vi "Interpolate SMPS distribution.vi"(8 "method":i32(ring)=3 items=["nearest", "linear", "spline", "cubic Hermite", "Lagrange"], 9 "samples":i32=10000, 10 "SMPS Sizes":dbl[](array[numeric])=[105.5, 109.4, 113.4, 117.6, 121.9, 126.3, 131.0, 135.8, 140.7, 145.9, 151.2, 156.8, 162.5, 168.5, 174.7, 181.1, 187.7, 194.6, 201.7, 209.1, 216.7, 224.7, 232.9, 241.4, 250.3, 259.5, 269.0, 278.8, 289.0, 299.6, 310.6, 322.0, 333.8, 346.0, 358.7, 371.8, 385.4, 399.5, 414.2, 429.4, 445.1, 461.4, 478.3, 495.8, 514.0, 532.8, 552.3, 572.5, 593.5, 615.3, 637.8, 661.2, 685.4, 710.5, 736.5, 763.5, 791.5], 11 "Concentration":dbl[](array[numeric])=[0.0, 0.0, 0.0, 0.0, 0.0, 0.0, 0.0, 0.0, 0.0, 0.0, 0.0, 0.0, 0.0, 0.0, 0.0, 0.0, 0.0, 0.0, 0.0, 0.0, 0.0, 0.0, 0.0, 0.0, 0.0, 0.0, 0.0, 0.0, 0.0, 0.0, 0.0, 0.0, 0.0, 0.0, 0.0, 0.0, 0.0, 0.0, 0.00157646, 0.0185973, 0.0849944, 0.192093, 0.275242, 0.234884, 0.133371, 0.0469575, 0.0107273, 0.00146543, 9.21708e-05, 0.0, 0.0, 0.0, 0.0, 0.0, 0.0, 0.0, 0.0]) -> (1 "DeltaX":dbl=8.752859881644426e-05, 2 "xi used":dbl[](array[numeric]), 3 "yi":dbl[](array[numeric]))   [LabVIEW 2013]
doc: "Interpolates SMPS distribution according to the number of sizes needed"
uses:
  <vilib>/Analysis/1siggen.llb/Ramp Pattern by Samples.vi
  <vilib>/gmath/NI_Gmath.lvlib
  <vilib>/Analysis/NI_AALBase.lvlib
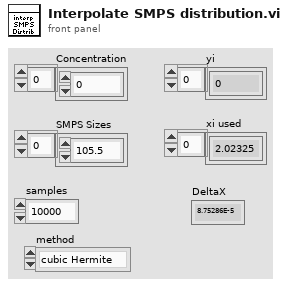
[diagram p1: front panel]
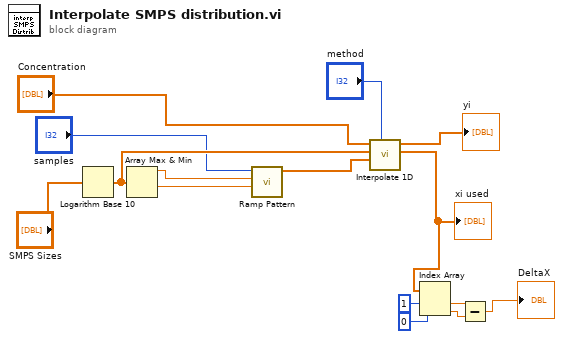
[diagram p0: block diagram]
diagram:
  n1 = Logarithm Base 10(1:"SMPS Sizes") -> (0:w13:dbl[])
  n2 = Array Max & Min(array=w13) -> (max value=w8:dbl, min value=w9:dbl)  [unwired: 2 out]
  n3 = call-poly <vilib>:"Ramp Pattern.vi"("start"=w9, "end"=w8, "samples"="samples") -> ("Ramp Pattern"=w11:dbl[])  [unwired: 7 in, 1 out]
  n4 = call <vilib>:"Interpolate 1D.vi"("method"="method", "xi"=w11, "X"=w13, "Y"="Concentration") -> ("xi used"=w7:dbl[], "yi"=→"yi":dbl[])  [unwired: 5 in, 1 out]
  "xi used" <- w7
  n5 = Index Array(array=w7, index #1=1 ("index"), index #2=0 ("index")) -> (element #1=w4:dbl, element #2=w3:dbl)
  n6 = Subtract(x=w4, y=w3) -> (x-y=→"DeltaX":dbl)
